vi "Linear Interp Resampler.vi"(4 "Single Sided FFT":bool, 5 "interp factor":i32=2, 6 "trunc interp data?":bool, 7 "Interp Type":i32(ring)=1 items=["nearest", "linear", "spline", "cubic Hermite", "Lagrange"], 8 "Window?":bool, 9 "forward FFT":bool, 10 "K-Data":dbl[](array[numeric]), 11 "OCT Data":dbl[](array[numeric])) -> (0 "Locations Used":dbl[](array[numeric]) format="%_6g", 2 "Interpolated Spectrum":cdb[](array[numeric]), 3 "Interpolated Data":dbl[](array[numeric]) format="%_6g")   [LabVIEW 2012]
uses:
  <vilib>/Analysis/4window.llb/windowTd.ctl
  <vilib>/Analysis/1siggen.llb/Ramp Pattern by Delta.vi
  <vilib>/Analysis/0measdsp.llb/Scaled Time Domain Window (DBL).vi
  <vilib>/Analysis/2dsp.llb/Inverse Complex FFT.vi
  <vilib>/Analysis/2dsp.llb/Real FFT.vi
  <vilib>/Analysis/NI_AALBase.lvlib
  <vilib>/gmath/NI_Gmath.lvlib
  <vilib>/Analysis/NI_AALPro.lvlib
panel:
  out "error":i32
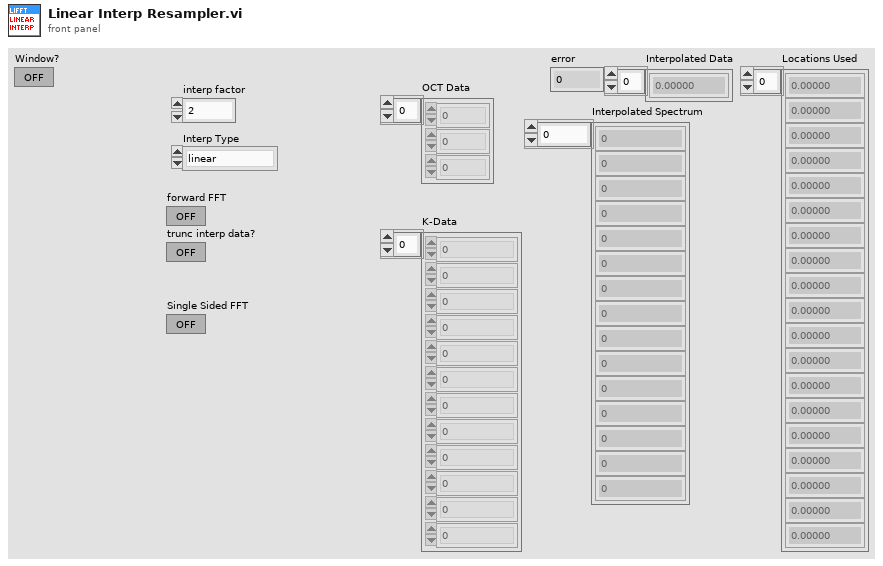
[diagram p1: front panel]
types:
  T1 = typedef "NI_AALPro.lvlib/windowTd.ctl" = u32
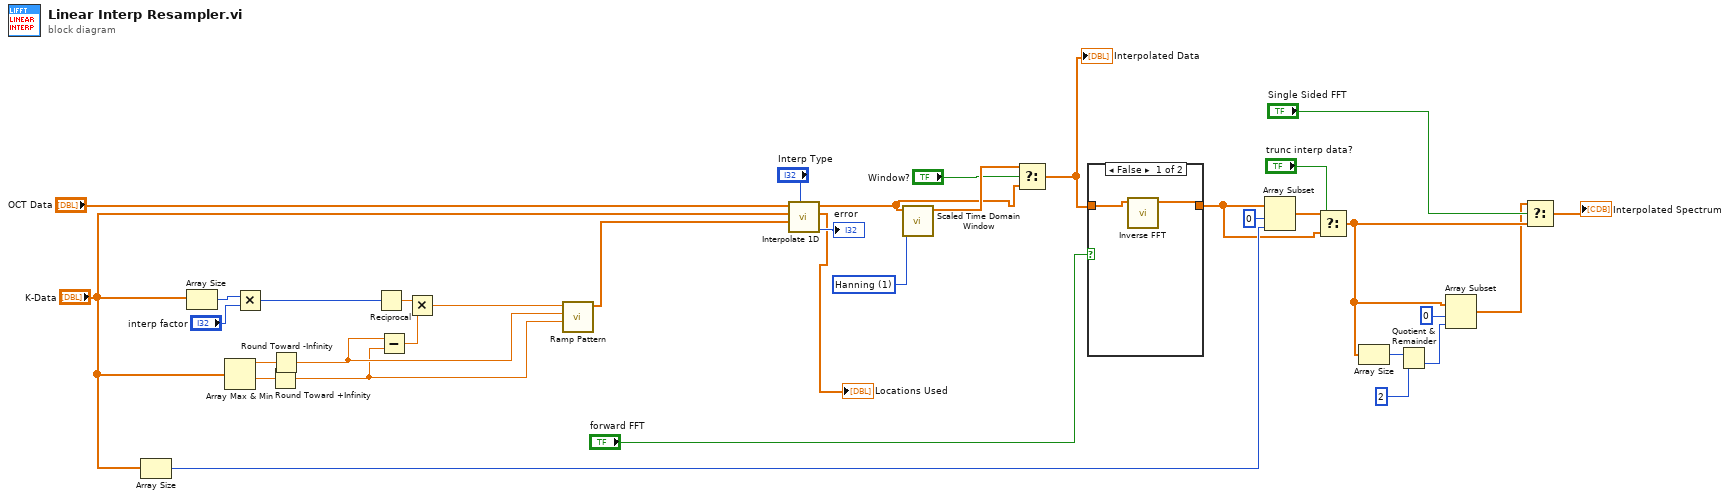
[diagram p0: block diagram]
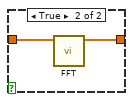
[diagram p2: hidden frame]
diagram:
  w19 = T1 1 items=["Rectangle"=0, "Hanning"=1, "Hamming"=2, "Blackman-Harris"=3, "Exact Blackman"=4, "Blackman"=5, "Flat Top"=6, "4 Term B-Harris "=7, "7 Term B-Harris"=8, "Low Sidelobe"=9, "Blackman Nuttall"=11, "Triangle"=30, "Bartlett-Hanning"=31, "Bohman"=32, "Parzen"=33, "Welch"=34, "Kaiser"=60, "Dolph-Chebyshev"=61, "Gaussian"=62] ("window")
  n1 = Array Size(array="K-Data") -> (size(s)=w24:i32)
  n2 = Array Size(array="K-Data") -> (size(s)=w32:i32)
  n3 = Array Max & Min(array="K-Data") -> (max value=w35:dbl, min value=w27:dbl)  [unwired: 2 out]
  n4 = Multiply(x=w32, y="interp factor") -> (x*y=w33:i32)
  n5 = Round Toward +Infinity(x=w27) -> (ceil(x): smallest int >= x=w9:dbl)
  n6 = Round Toward -Infinity(1:w35) -> (0:w10:dbl)
  n7 = Reciprocal(x=w33) -> (1/x=w34:dbl)
  n8 = Subtract(x=w10, y=w9) -> (x-y=w7:dbl)
  n9 = Multiply(x=w34, y=w7) -> (x*y=w6:dbl)
  n10 = call-poly <vilib>:"Ramp Pattern.vi"("start"=w9, "end"=w10, "delta"=w6) -> ("Ramp Pattern"=w5:dbl[])  [unwired: 6 in, 2 out]
  n11 = call <vilib>:"Interpolate 1D.vi"("method"="Interp Type", "xi"=w5, "X"="K-Data", "Y"="OCT Data") -> ("error"=→"error":i32, "xi used"=→"Locations Used":dbl[], "yi"=w3:dbl[])  [unwired: 5 in]
  n12 = call-poly <vilib>:"Scaled Time Domain Window.vi"("window"=w19, "X"=w3) -> ("Windowed X"=w4:dbl[])  [unwired: 7 in, 2 out]
  n13 = Select(t=w4, s="Window?", f=w3) -> (s? t:f=w2:dbl[])
  "Interpolated Data" <- w2
  n14 = case shown="False" "forward FFT" {
    tunnel: w2 -> [w37 w39]
    tunnel: [w36 w38] -> w20
    frame False {
      n15 = call-poly <vilib>:"Inverse FFT.vi"("FFT {X}"=w37) -> ("X"=w36:cdb[])  [unwired: 9 in, 1 out]
    }
    frame True {
      n16 = call-poly <vilib>:"FFT.vi"("X"=w39) -> ("FFT {X}"=w38:cdb[])  [unwired: 9 in, 1 out]
    }
  }
  n17 = Array Subset(array=w20, index=0, length=w24) -> (w22:cdb[])
  n18 = Select(t=w22, s="trunc interp data?", f=w20) -> (s? t:f=w12:cdb[])
  n19 = Array Size(array=w12) -> (size(s)=w15:i32)
  n20 = Quotient & Remainder(x=w15, y=2) -> (floor(x/y)=w13:i32)  [unwired: 1 out]
  n21 = Array Subset(array=w12, index=0, length=w13) -> (w11:cdb[])
  n22 = Select(t=w11, s="Single Sided FFT", f=w12) -> (s? t:f=→"Interpolated Spectrum":cdb[])
